vi "CLSUIP_UserScripting.vi"(8 "error in":errorcluster, 10 "VI Refnum in":refnum<vi>, 11 "VIRetooler":refnum<class "VIRetooler.lvclass">) -> (0 "error out":errorcluster, 3 "VIRetooler out":refnum<class "VIRetooler.lvclass">)   [LabVIEW 2021, in "MemberVICreation.lvlib" / "VIRetooler.lvclass"]
doc: "This VI does nothing. It provides an opportunity for users to add scripting code of their own to modify the retooling process even if they do not have the password to the VIs in the retooling process. Each overriding class should call out to an empty subVI, one that is not a member of the class, that users can edit to put in their own scripting behavior."
uses:
  <resource>/Framework/Providers/LVClassLibrary/NewAccessors/VIRetooler/VIRetooler.lvclass
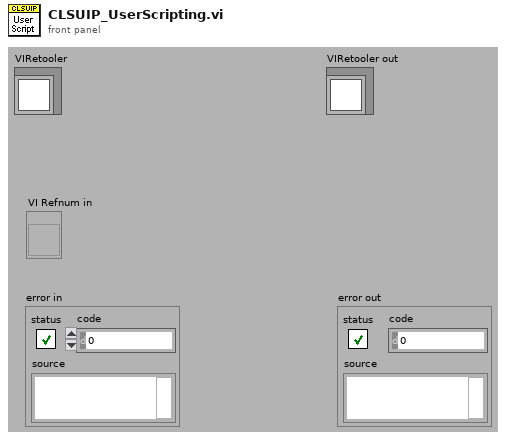
[diagram p1: front panel]
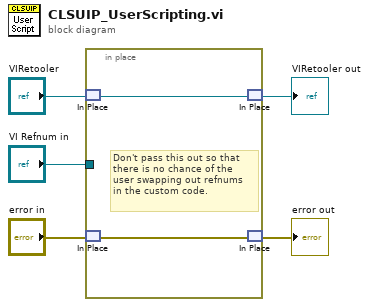
[diagram p0: block diagram]
diagram:
  n1 = in-place {
    in-place-border: "VI Refnum in" -> [_]
    # "Don't pass this out so that\nthere is no chance of the \nuser swapping out refnums\nin the custom code."
    n2 = in-place-match #1("VIRetooler") -> (w6:refnum<class "VIRetooler.lvclass">)
    n3 = in-place-match #2("error in") -> (w7:errorcluster)
    n4 = in-place-match #1(w6) -> (→"VIRetooler out":refnum<class "VIRetooler.lvclass">)
    n5 = in-place-match #2(w7) -> (→"error out":errorcluster)
  }
